vi "LVClasse_Phase Write SurfaceFloatWithPupil.vi"(8 "error in (no error)":errorcluster, 10 "SurfaceFloatWithPupil":i32, 11 "Phase in":refnum<class "Phase.lvclass">) -> (0 "error out":errorcluster, 3 "Phase out":refnum<class "Phase.lvclass">)   [LabVIEW 2020, in "Phase.lvclass"]
uses:
  Phase.lvclass
  Phase.lvclass/Phase.ctl
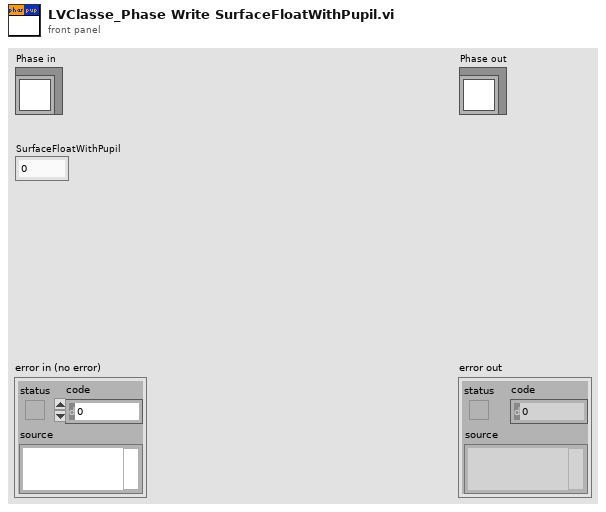
[diagram p1: front panel]
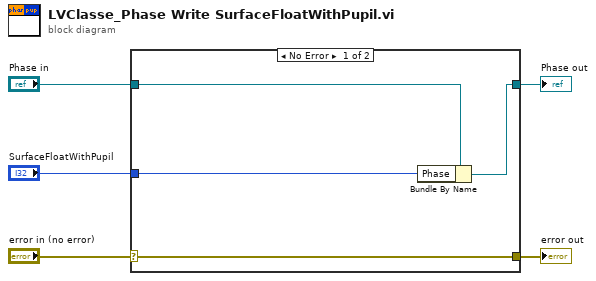
[diagram p0: block diagram]
diagram:
  n1 = case shown="No Error" "error in (no error)" {
    selector: "error in (no error)" -> [w9 w10]
    tunnel: [w9 w10] -> w4
    tunnel: [w7 w11] -> w2
    tunnel: "Phase in" -> [w8 w11]
    tunnel: "SurfaceFloatWithPupil" -> [w6 _]
    frame No Error {
      n2 = Bundle By Name(cluster=w8, "Phase"=w6) -> (w7:refnum<class "Phase.lvclass">)
    }
    frame Error {
    }
  }
  "error out" <- w4
  "Phase out" <- w2
